vi "SortRunCluster.vi"(1 "Array":T1(array[cluster])) -> (0 "output array":T1(array[cluster]))   [LabVIEW 2018]
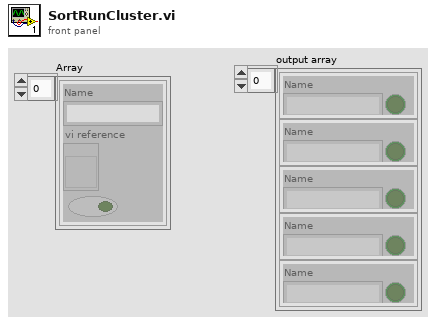
[diagram p1: front panel]
types:
  T1 = cluster{"Name":string, "vi reference":refnum<vi>, bool}[]
  T2 = cluster{"Name":string, "vi reference":refnum<vi>, "Running?":bool}[]
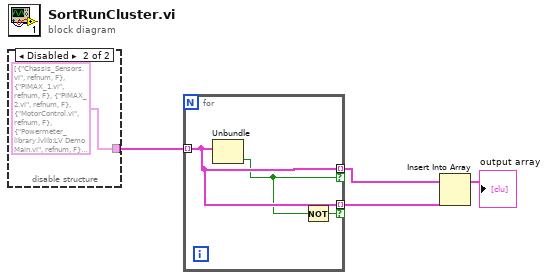
[diagram p0: block diagram]
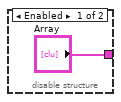
[diagram p2: hidden frame]
diagram:
  n1 = disable-structure shown="Disabled" {
    disable-tunnel: ["Array" T2 [{"Name"="Chassis_Sensors.vi", "vi reference"=refnum, "Running?"=FALSE}, {"Name"="PIMAX_1.vi", "vi reference"=refnum, "Running?"=FALSE}, {"Name"="PIMAX_2.vi", "vi reference"=refnum, "Running?"=FALSE}, {"Name"="MotorControl.vi", "vi reference"=refnum, "Running?"=FALSE}, {"Name"="Powermeter_library.lvlib:LV Demo Main.vi", "vi reference"=refnum, "Running?"=FALSE}, {"Name"="Multiplexer.vi", "vi reference"=refnum, "Running?"=FALSE}, {"Name"="NIR.vi", "vi reference"=refnum, "Running?"=FALSE}, {"Name"="Vis.vi", "vi reference"=refnum, "Running?"=FALSE}] ("Instruments")] -> w4
    frame Enabled {
    }
    frame Disabled {
    }
  }
  n2 = for {
    tunnel: w4 -> [w9] mode=indexing
    tunnel: [w9] -> w3 mode=indexing if=w8
    tunnel: [w9] -> w2 mode=indexing if=w7
    n3 = Unbundle(w9) -> (w8:bool)  [unwired: 2 out]
    n4 = Not(x=w8) -> (.not. x?=w7:bool)
  }
  n5 = Insert Into Array(array=w3, new element=w2) -> (→"output array":T1)  [unwired: 1 in]
